vi "HXG2_LinearInterp_EvapPV.vi"(7 "CFM":dbl, 10 "Tair  °F":dbl, 11 "Evap Target Delta (-°F) in":cluster{"m":dbl, "b":dbl}) -> (3 "Evap Target (F)":dbl)   [LabVIEW 2012]
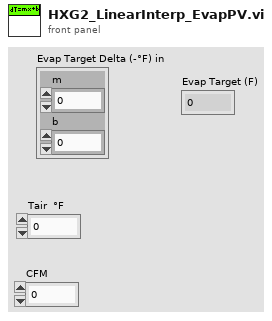
[diagram p1: front panel]
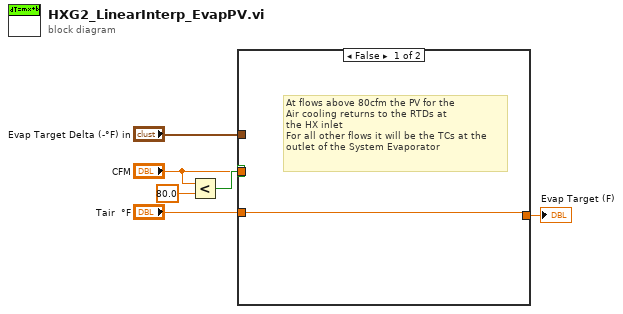
[diagram p0: block diagram]
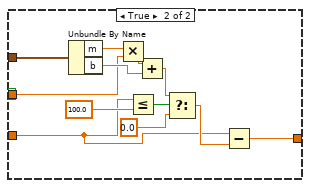
[diagram p2: hidden frame]
diagram:
  n1 = Less?(x="CFM", y=80.0) -> (x < y?=w3:bool)
  n2 = case shown="False" w3 {
    tunnel: "Evap Target Delta (-°F) in" -> [_ w12]
    tunnel: "Tair  °F" -> [w7 w10]
    tunnel: [w7 w9] -> w4
    tunnel: "CFM" -> [_ w8]
    frame False {
      # "At flows above 80cfm the PV for the \nAir cooling returns to the RTDs at \nthe HX inlet\nFor all other flows it will be the TCs at the \noutlet of the System Evaporator"
    }
    frame True {
      n3 = Unbundle By Name(w12) -> ("m"=w13:dbl, "b"=w14:dbl)
      n4 = Multiply(x=w13, y=w8) -> (x*y=w15:dbl)
      n5 = Less Or Equal?(x=w10, y=100.0) -> (x <= y?=w17:bool)
      n6 = Add(x=w15, y=w14) -> (x+y=w18:dbl)
      n7 = Select(t=w18, s=w17, f=0.0) -> (s? t:f=w11:dbl)
      n8 = Subtract(x=w10, y=w11) -> (x-y=w9:dbl)
    }
  }
  "Evap Target (F)" <- w4
